vi "engine.executor.vi"(6 "Enable Queues (T)":bool=TRUE, 8 "error":errorcluster, 9 "Index(-1: All)":i32=-1, 10 "clk (NaN)":dbl=nan, 11 "Procs in":cluster{"Procedure":variant[]}[](array[cluster])) -> (0 "Error":errorcluster, 2 "runtime[ms]":u32, 3 "Procs out":cluster{"proc out":variant[]}[](array[cluster]), 4 "ErrorProcs out":T1(array[cluster]))   [LabVIEW 2024]
uses:
  controls/state-engine.ctl
  engine.prestep.vi
  engine-step-function.vi
  engine.poststep.calc.vi
  globals/globals-engine.vi
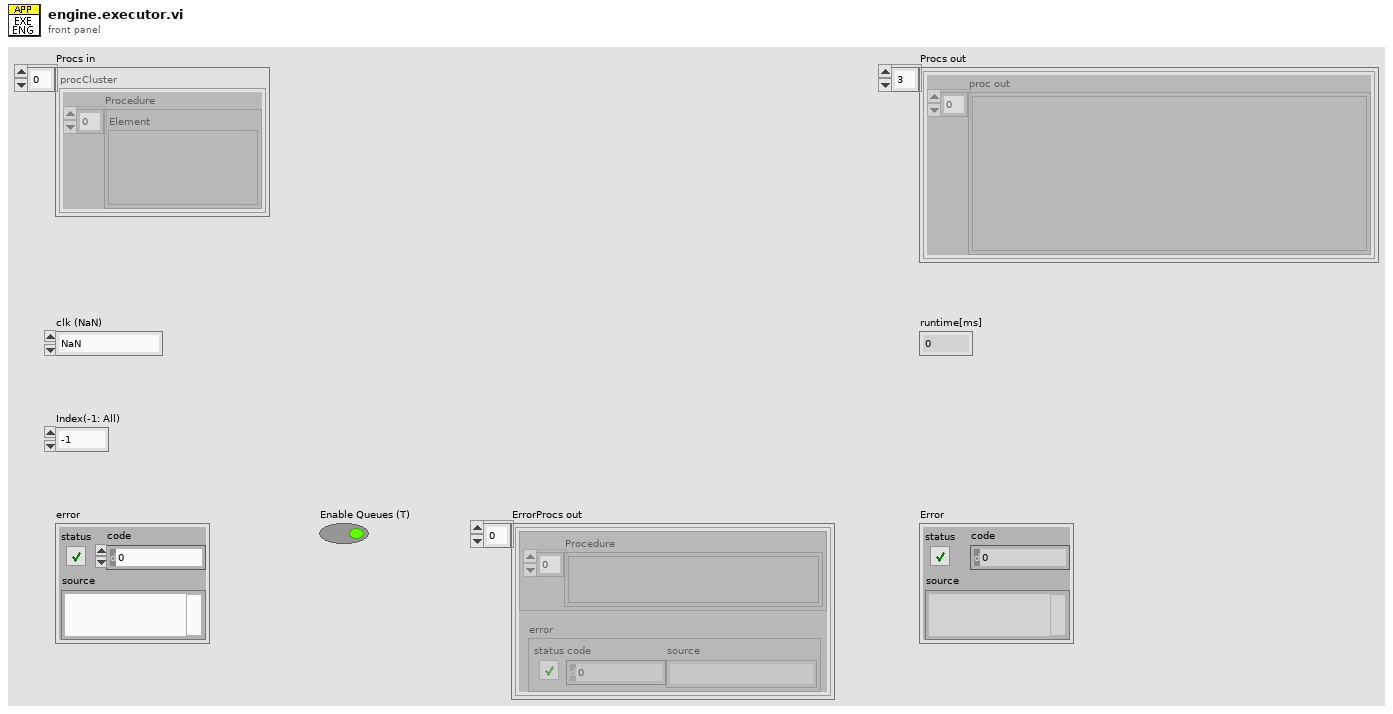
[diagram p1: front panel]
types:
  T1 = cluster{cluster{"Procedure":variant[]}, "error":errorcluster}[]
  T2 = typedef "state-engine.ctl" = enum16{"ENG.NO-OP", "ENG.START", "ENG.STOP", "ENG.EXECUTE", "ENG.STATUS", "ENG.EXTERNAL-CALL", "ENG.INIT", "ENG.INIT.VARS", "ENG.INIT.SERIAL", "ENG.LOAD", "ENG.LOAD.SINGLE", "ENG.LOAD.MODULE", "ENG.LOAD.RELOAD", "ENG.LOAD.UNLOAD", "ENG.IO.LOAD", "ENG.IO.SAVE", "ENG.PROC.RELOAD-BY-NAME", "ENG.PROC.START", "ENG.PROC.STOP", "ENG.PROC.INSERT-STEPS", "ENG.PROC.ISRUNNING", "ENG.PROC.PRESET", "ENG.PROC.STATUS", "ENG.PRINT-USER-MSG", "ENG.RIO.SNAPSHOT", "ENG.RIO.AIN-SNAPSHOT-CALIB", "ENG.RIO.DOUT-BY-ADDR", "ENG.RIO.DOUT-BY-NAME", "ENG.RIO.RFS-DELAY-SET-X1", "ENG.RIO.RFS-DELAY-SET-X8", "ENG.RIO.RFS-CYCLES-SET", "ENG.RIO.RFS-CYCLES-GET", "ENG.RIO.RFS-ENABLE", "ENG.EXIT"}
  T3 = typedef "state-logger.ctl" = enum16{"LOG.NO_OP", "LOG.INIT", "LOG.INIT.NTR-FLOW", "LOG.EXIT", "LOG.CATCH", "LOG.PARSE.OCS", "LOG.UPDATE.SELECTORS", "LOG.UPDATE.IRR", "LOG.SNAPSHOT.PROC", "LOG.SNAPSHOT"}
  T4 = cluster{"procCluster":cluster{"Procedure":variant[]}, "error out":errorcluster}
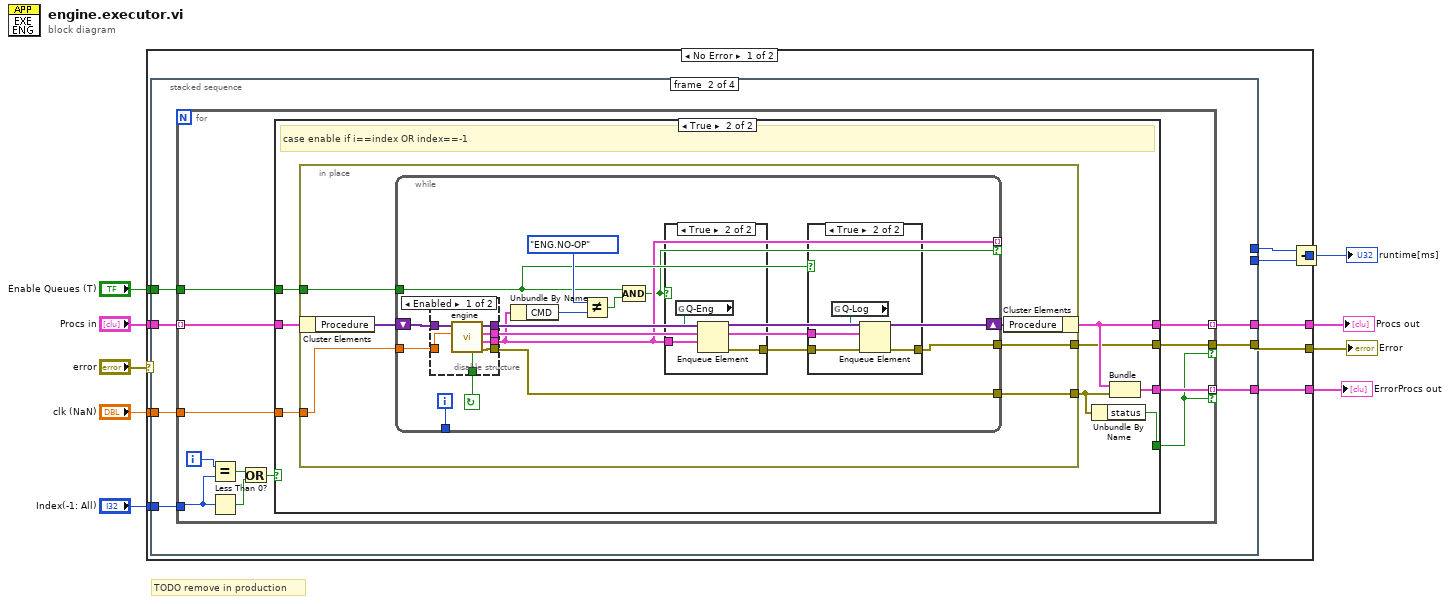
[diagram p0: block diagram]
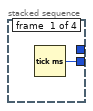
[diagram p2: hidden frame]
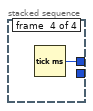
[diagram p8: hidden frame]
diagram:
  # "TODO remove in production"
  n1 = case shown="No Error" "error" {
    selector: "error" -> [_ w88]
    tunnel: [w19 _] -> w9
    tunnel: [w16 w87] -> w8
    tunnel: "Procs in" -> [w15 w87]
    tunnel: "Enable Queues (T)" -> [w14 _]
    tunnel: [w13 _] -> w5
    tunnel: "clk (NaN)" -> [w12 _]
    tunnel: [w11 w88] -> w3
    tunnel: "Index(-1: All)" -> [w10 _]
    frame No Error {
      n2 = stacked-sequence {
        tunnel: w15 -> [_ w27 _ _]
        tunnel: [_ w26 _ _] -> w16
        tunnel: [w20 _ _ _] -> w17
        tunnel: [_ _ _ w86] -> w18
        tunnel: w14 -> [_ w25 _ _]
        tunnel: [_ w24 _ _] -> w13
        tunnel: w12 -> [_ w23 _ _]
        tunnel: [_ w22 _ _] -> w11
        tunnel: w10 -> [_ w21 _ _]
        frame #0 {
          n3 = Tick Count (ms)() -> (millisecond timer value=w20:u32)
        }
        frame #1 {
          n4 = for {
            tunnel: [w36] -> w26 mode=indexing
            tunnel: w27 -> [w38] mode=indexing
            tunnel: w25 -> [w39]
            tunnel: [w37] -> w24 mode=indexing if=w28
            tunnel: w23 -> [w35]
            tunnel: [w29] -> w22 if=w28
            tunnel: w21 -> [w31]
            i -> [w34]
            n5 = Equal?(x=w34, y=w31) -> (x = y?=w33:bool)
            n6 = Less Than 0?(x=w31) -> (x < 0?=w30:bool)
            n7 = Or(x=w33, y=w30) -> (x .or. y?=w32:bool)
            n8 = case shown="True" w32 {
              tunnel: w39 -> [_ w48]
              tunnel: w38 -> [w40 w47]
              tunnel: [_ w46] -> w37
              tunnel: [w40 w45] -> w36
              tunnel: w35 -> [_ w44]
              tunnel: [_ w41] -> w28
              tunnel: [_ w43] -> w29
              frame False {
              }
              frame True {
                # "case enable if i==index OR index==-1"
                n9 = in-place {
                  in-place-border: [w51] -> w43
                  in-place-border: w48 -> [w50]
                  in-place-border: w44 -> [w53]
                  in-place-border: [w49] -> w42
                  n10 = in-place-cluster #1(w47) -> ("Procedure"=w52:variant[])
                  n11 = while {
                    tunnel: w53 -> [w68]
                    tunnel: [w57] -> w51
                    tunnel: w50 -> [w62]
                    tunnel: [w61] -> w49
                    shift-right: [w69] -> w54
                    shift-left: w52 -> [w67]
                    tunnel: [w58] -> _
                    tunnel: [w56] -> _ mode=indexing if=w55
                    i -> [w58]
                    stop <- w59 continue-if-true
                    n12 = disable-structure shown="Enabled" {
                      disable-tunnel: [w76 w77] -> w69
                      disable-tunnel: w68 -> [w75 _]
                      disable-tunnel: w67 -> [w74 w77]
                      disable-tunnel: [w73 _] -> w56
                      disable-tunnel: [w72 _] -> w63
                      disable-tunnel: [w71 _] -> w61
                      disable-tunnel: [w70 _] -> w59
                      frame Enabled {
                        n13 = call "engine.vi"("clk (NaN)"=w75, "Procedure in"=w74) -> ("error out"=w71:errorcluster, "cmdEng"=w73:cluster{"CMD":T2, "data":variant}, "Q-Log Command"=w72:cluster{"data":variant, "Enum":T3}, "Procedure out"=w76:variant[], "Continue?"=w70:bool)  [unwired: 5 in]
                      }
                      frame Disabled {
                      }
                    }
                    n14 = Unbundle By Name(w56) -> ("CMD"=w65:T2)
                    n15 = Not Equal?(x=state-engine."ENG.NO-OP" ("CMD"), y=w65) -> (x != y?=w64:bool)
                    n16 = Compound Arithmetic op=AND(w62, w64) -> (w55:bool)
                    n17 = case shown="True" w55 {
                      tunnel: w56 -> [_ w85]
                      tunnel: [_ w84] -> w60
                      frame False {
                      }
                      frame True {
                        n18 = global read "globals-engine.vi" "Q-Eng"() -> (w83:refnum<queue>)
                        n19 = Enqueue Element(queue=w83, element=w85) -> (error out=w84:errorcluster)  [unwired: 2 in, 2 out]
                      }
                    }
                    n20 = case shown="True" w62 {
                      tunnel: [w78 w82] -> w57
                      tunnel: w63 -> [_ w80]
                      tunnel: w60 -> [w78 w79]
                      frame False {
                      }
                      frame True {
                        n21 = global read "globals-engine.vi" "Q-Log"() -> (w81:refnum<queue>)
                        n22 = Enqueue Element(queue=w81, element=w80, error in (no error)=w79) -> (error out=w82:errorcluster)  [unwired: 1 in, 2 out]
                      }
                    }
                  }
                  n23 = in-place-cluster #1("Procedure"=w54) -> (w45:cluster{"Procedure":variant[]})
                }
                n24 = Unbundle By Name(w42) -> ("status"=w41:bool)
                n25 = Bundle("procCluster"=w45, "error out"=w42) -> (w46:T4)  [unwired: 1 in]
              }
            }
          }
        }
        frame #2 {
        }
        frame #3 {
          n26 = Tick Count (ms)() -> (millisecond timer value=w86:u32)
        }
      }
      n27 = Subtract(x=w18, y=w17) -> (x-y=w19:u32)
    }
    frame Error {
    }
  }
  "runtime[ms]" <- w9
  "Error" <- w3
  "Procs out" <- w8
  "ErrorProcs out" <- w5
